vi "FindBlueSerializableTemplates.vi"(8 "error in (no error)":errorcluster, 10 "App Reference (this app)":refnum<vi>, 11 "LabVIEW Class Path":path) -> (0 "error out":errorcluster, 3 "BlueSerializableTemplate Paths":T1)   [LabVIEW 2019, in "BlueSerializationScripts.lvlib"]
uses:
  BlueSerializationScripts.lvlib
  BlueSerializableTemplatePaths.ctl
  BlueSerialProviderGlobal.vi
  <vilib>/Utility/error.llb/Error Cluster From Error Code.vi
  <vilib>/ErrorRing/Error Ring.xnode
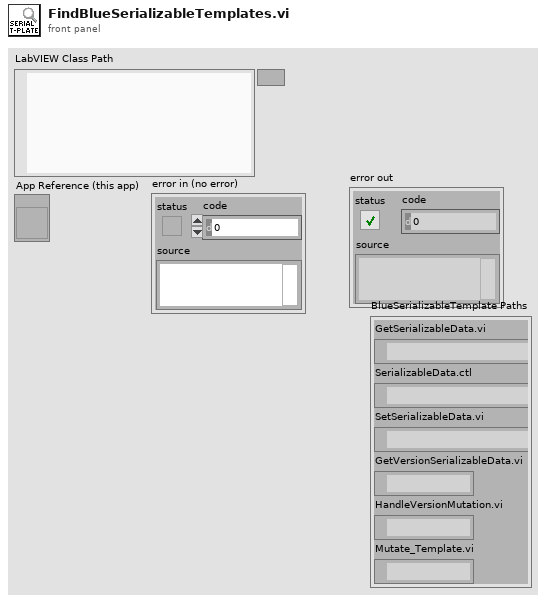
[diagram p1: front panel]
types:
  T1 = typedef "BlueSerializationScripts.lvlib/BlueSerializableTemplatePaths.ctl" = cluster{"GetSerializableData.vi":path, "SerializableData.ctl":path, "SetSerializableData.vi":path, "GetVersionSerializableData.vi":path, "HandleVersionMutation.vi":path, "Mutate_Template.vi":path}
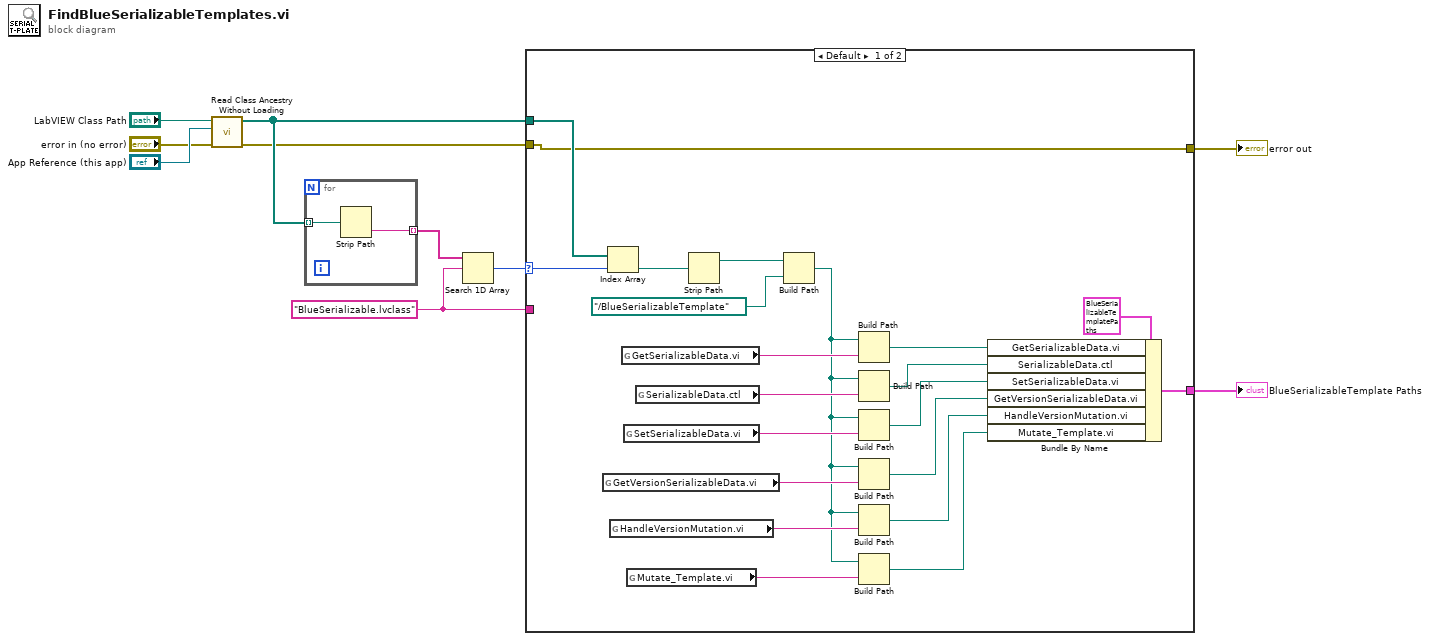
[diagram p0: block diagram]
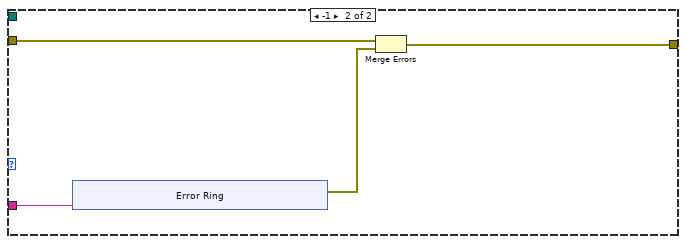
[diagram p2: hidden frame]
diagram:
  w4 = "BlueSerializable.lvclass" ("name")
  n1 = call <vilib>:"Read Class Ancestry Without Loading.vi"("error in (no error)"="error in (no error)", "App Reference (this app)"="App Reference (this app)", "LabVIEW Class Path"="LabVIEW Class Path") -> ("error out"=w3:errorcluster, "Class Ancestry"=w8:path[])  [unwired: 7 in]
  n2 = for {
    tunnel: w8 -> [w12] mode=indexing
    tunnel: [w11] -> w10 mode=indexing
    n3 = Strip Path(path=w12) -> (name=w11:string)  [unwired: 1 out]
  }
  n4 = Search 1D Array(1D array=w10, element=w4) -> (index of element=w9:i32)  [unwired: 1 in]
  n5 = case shown="Default" w9 {
    selector: w9 -> [w32 _]
    tunnel: w8 -> [w33 _]
    tunnel: w4 -> [_ w37]
    tunnel: w3 -> [w23 w36]
    tunnel: [w23 w34] -> w2
    tunnel: [w24 _] -> w1
    frame Default {
      n6 = global read "BlueSerialProviderGlobal.vi" "GetVersionSerializableData.vi"() -> (w19:string)
      n7 = Index Array(array=w33, index=w32) -> (element=w31:path)
      n8 = global read "BlueSerialProviderGlobal.vi" "HandleVersionMutation.vi"() -> (w18:string)
      n9 = global read "BlueSerialProviderGlobal.vi" "GetSerializableData.vi"() -> (w22:string)
      n10 = global read "BlueSerialProviderGlobal.vi" "SetSerializableData.vi"() -> (w20:string)
      n11 = global read "BlueSerialProviderGlobal.vi" "Mutate_Template.vi"() -> (w17:string)
      n12 = global read "BlueSerialProviderGlobal.vi" "SerializableData.ctl"() -> (w21:string)
      n13 = Strip Path(path=w31) -> (stripped path=w30:path)  [unwired: 1 out]
      n14 = Build Path(base path=w30, name or relative path=path "../BlueSerializableTemplate" ("stripped path")) -> (appended path=w16:path)
      n15 = Build Path(base path=w16, name or relative path=w22) -> (appended path=w27:path)
      n16 = Build Path(base path=w16, name or relative path=w21) -> (appended path=w26:path)
      n17 = Build Path(base path=w16, name or relative path=w20) -> (appended path=w25:path)
      n18 = Build Path(base path=w16, name or relative path=w19) -> (appended path=w15:path)
      n19 = Build Path(base path=w16, name or relative path=w18) -> (appended path=w14:path)
      n20 = Build Path(base path=w16, name or relative path=w17) -> (appended path=w13:path)
      n21 = Bundle By Name(cluster=T1 {"GetSerializableData.vi"=path "", "SerializableData.ctl"=path "", "SetSerializableData.vi"=path "", "GetVersionSerializableData.vi"=path "", "HandleVersionMutation.vi"=path "", "Mutate_Template.vi"=path ""} ("BlueSerializableTemplate Paths"), "GetSerializableData.vi"=w27, "SerializableData.ctl"=w26, "SetSerializableData.vi"=w25, "GetVersionSerializableData.vi"=w15, "HandleVersionMutation.vi"=w14, "Mutate_Template.vi"=w13) -> (w24:T1)
    }
    frame -1 {
      n22 = xnode "Error Ring"("parameter 0"=w37) -> ("error out"=w35:errorcluster)
      n23 = Merge Errors(w36, w35) -> (w34:errorcluster)
    }
  }
  "error out" <- w2
  "BlueSerializableTemplate Paths" <- w1
